vi "shortURL (SubVI).vi"(1 "LON":string, 2 "LAT":string) -> (0 "before substring":string)   [LabVIEW 2012]
panel:
  out "result string":string
  out "HTML as string":string
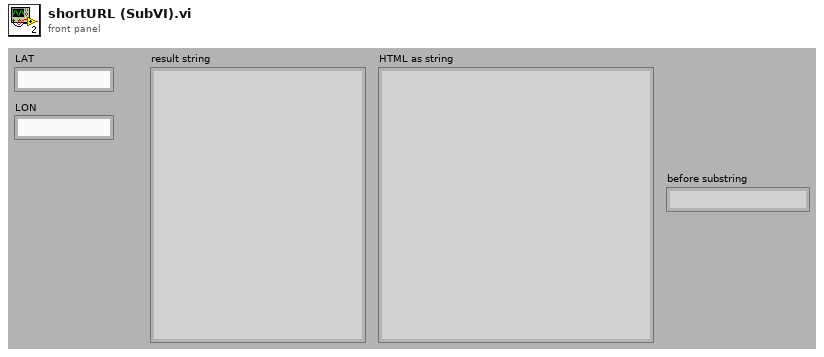
[diagram p1: front panel]
types:
  T1 = enum16{"Read", "Write", "ReadWrite", "BufferedRead", "BufferedReadWrite"}
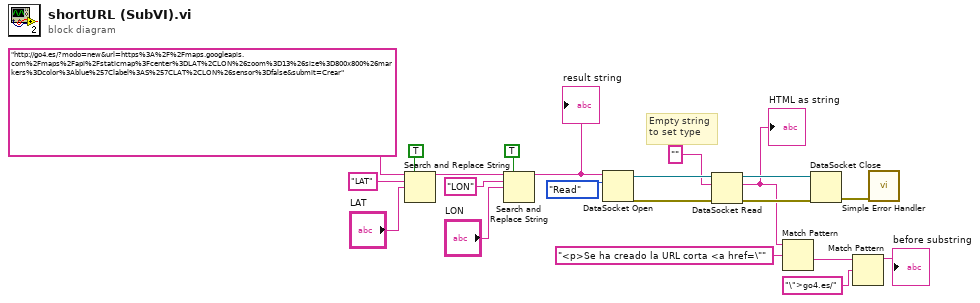
[diagram p0: block diagram]
diagram:
  # "Empty string\nto set type"
  n1 = Search and Replace String(replace all?=TRUE ("replace all? (F)"), input string="http://go4.es/?modo=new&url=https%3A%2F%2Fmaps.googleapis.com%2Fmaps%2Fapi%2Fstaticmap%3Fcenter%3DLAT%2CLON%26zoom%3D13%26size%3D800x800%26markers%3Dcolor%3Ablue%257Clabel%3AS%257CLAT%2CLON%26sensor%3Dfalse&submit=Crear" ("URL"), search string="LAT", replace string="LAT") -> (result string=w6:string)  [unwired: 4 in, 3 out]
  n2 = Search and Replace String(replace all?=TRUE ("replace all? (F)"), input string=w6, search string="LON", replace string="LON") -> (result string=w3:string)  [unwired: 4 in, 3 out]
  "result string" <- w3
  n3 = DataSocket Open(10:T1."Read" ("mode"), 11:w3) -> (0:w18:errorcluster, 3:w21:refnum<k13>)  [unwired: 2 in]
  n4 = DataSocket Read(8:w18, 10:"", 11:w21) -> (0:w19:errorcluster, 2:w14:string, 3:w20:refnum<k13>)  [unwired: 2 in, 4 out]
  "HTML as string" <- w14
  n5 = Match Pattern(string=w14, regular expression="<p>Se ha creado la URL corta <a href=\"") -> (after substring=w12:string)  [unwired: 1 in, 3 out]
  n6 = DataSocket Close(8:w19, 11:w20) -> (0:w15:errorcluster)  [unwired: 1 in, 1 out]
  n7 = Match Pattern(string=w12, regular expression="\">go4.es/") -> (before substring=→"before substring":string)  [unwired: 1 in, 3 out]
  n8 = call <vilib>:"Simple Error Handler.vi"("error in (no error)"=w15) -> ()  [unwired: 4 in, 5 out]
